vi "Fetch Power Measurement CCDF Statistic Results.vi"(8 "error in (no error)":errorcluster, 9 "Instance (1)":i32=1, 11 "VISA resource name":refnum<visa-resource-name>) -> (0 "error out":errorcluster, 1 "Average":dbl format="%^.3e", 2 "Reliability":i32, 3 "VISA resource name out":refnum<visa-resource-name>, 4 "Maximum":dbl format="%^.3e", 5 "PAR":dbl format="%^.3e", 6 "Index":i32)   [LabVIEW 2020, in "Rohde&Schwarz CMXP GPRF.lvlib"]
doc: "Returns the power results in \"Statistic\" evaluation mode (rscmwgprf Configure Power Measurement Result Mode.vi).\n\nAttribute:\nRSCMXPGPRF_ATTR_FETCH_POWER_MEASUREMENT_CCDF_STATISTIC_RESULTS\n\nRemote-control command:\nFETCh:GPRF:MEAS<i>:POWer:CCDF:POWer?"
uses:
  <instrlib>/Rohde&Schwarz CMXP GPRF/Rohde&Schwarz CMXP GPRF.lvlib
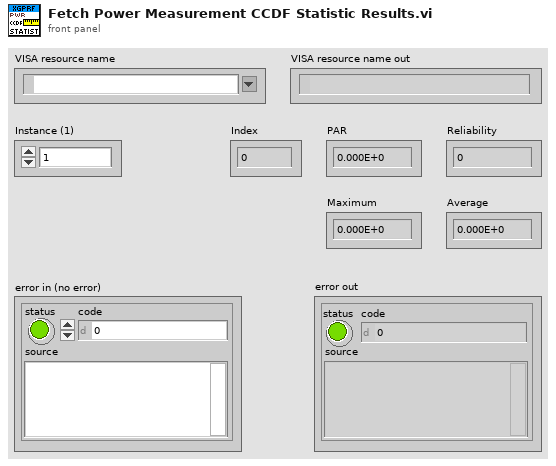
[diagram p1: front panel]
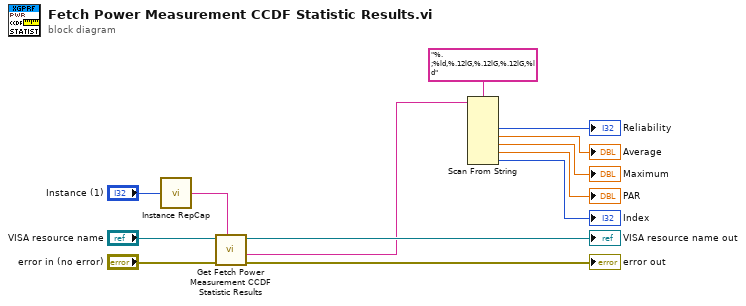
[diagram p0: block diagram]
diagram:
  n1 = call <instrlib>:"Instance RepCap.vi"("Instance in"="Instance (1)") -> ("Instance out"=w8:string)
  n2 = call "Get Fetch Power Measurement CCDF Statistic Results"("Repeated Capabilities"=w8, "error in (no error)"="error in (no error)", "instrument handle"="VISA resource name") -> ("error out"=→"error out":errorcluster, "Fetch Power Measurement CCDF Statistic Results"=w5:string, "instrument handle out"=→"VISA resource name out":refnum<visa-resource-name>)  [unwired: 6 in]
  n3 = Scan From String(format string="%.;%ld,%.12lG,%.12lG,%.12lG,%ld", input string=w5) -> (output 1=→"Reliability":i32, output 2=→"Average":dbl, output 3=→"Maximum":dbl, output 4=→"PAR":dbl, output 5=→"Index":i32)  [unwired: 7 in, 3 out]
